vi "main.vi"(4 "Input":string="((sin(((20+35) / exp(4))) + cos(256))^(1/5))") -> (1 "Result":string)   [LabVIEW 2020]
panel:
  # "Impemented functions:\n* / + - ^\nsin cos tg ctg\nexp"
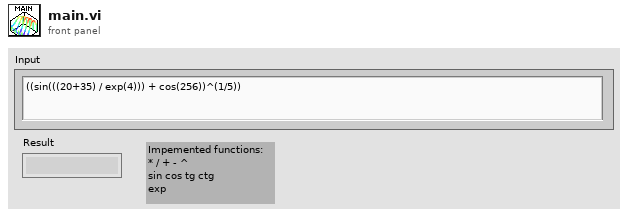
[diagram p1: front panel]
types:
  T1 = typedef "SplittedString.ctl" = string[]
  T2 = typedef "SplittedStringTokens.ctl" = T3[]
  T3 = typedef "Classes.ctl" = enum16{"Undefined", "Left paren", "Right paren", "Number", "Operator", "High level function", "Variable", "End of expression"}
  T4 = typedef "Tree Map.lvlib/Tree Map Data.ctl" = map{string, cluster{"Child Paths Set":set{string}, "Name":string, "Data":string, "Attributes":map{string, string}}}
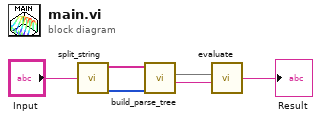
[diagram p0: block diagram]
diagram:
  n1 = call "split_string.vi"("String"="Input") -> ("Splitted string"=w5:T1, "Splitted string tokens"=w4:T2)  [unwired: 8 in]
  n2 = call "build_parse_tree.vi"("Splitted string tokens"=w4, "Splitted string"=w5) -> ("Root Path"=w2:string, "Tree Map Out"=w3:T4)  [unwired: 7 in]
  n3 = call "evaluate.vi"("Parse Tree In"=w3, "Node Path"=w2) -> ("Result"=→"Result":string)  [unwired: 6 in]
